vi "Get as Path.vi"(8 "error in (no error)":errorcluster, 10 "Name Array":string[](array[string]), 11 "JSON Scalar in":refnum<class "JSON Value.lvclass">) -> (0 "error out":errorcluster, 2 "path":path, 3 "JSON Scalar out":refnum<class "JSON Value.lvclass">)   [LabVIEW 2011, in "JSON Scalar.lvclass"]
doc: "Converts a <b>JSON Value</b> into a <b>File Path</b>.\n\nCopyright 2012 James David Powell, Shaun Rumbell and Ton Plomp\nMore information on http://lavag.org/topic/16217-cr-json-labview"
uses:
  JSON Scalar.lvclass
  JSON Value/JSON Value.lvclass
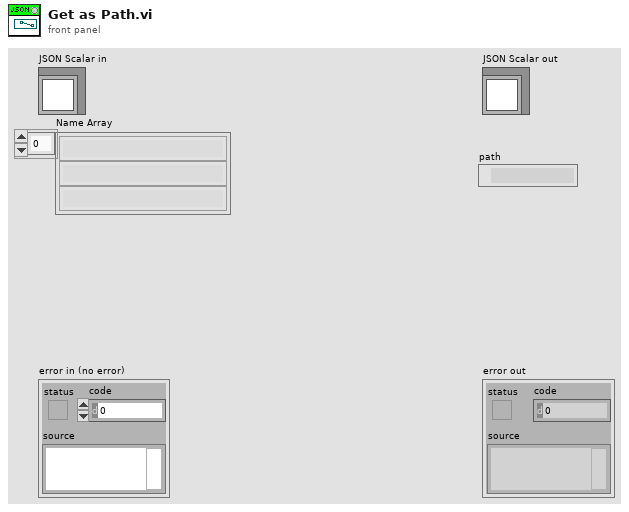
[diagram p1: front panel]
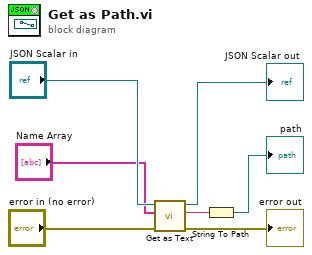
[diagram p0: block diagram]
diagram:
  n1 = call "Get as Text.vi"("error in (no error)"="error in (no error)", "Name Array"="Name Array", "JSON Scalar in"="JSON Scalar in") -> ("error out"=→"error out":errorcluster, "LabVIEW Text"=w2:string, "JSON Scalar out"=→"JSON Scalar out":refnum<class "JSON Value.lvclass">)  [unwired: 6 in]
  n2 = String To Path(string=w2) -> (path=→"path":path)
